vi "sub vi - AI USB4704 (3)  Create Task v2.vi"(0 "Task In 0":dbl, 5 "Task In 1":dbl, 7 "Task In 2":dbl) -> (4 "TASK USB 0":i32, 6 "TASK USB 1":i32, 8 "TASK USB 2":i32, 14 "AI Task Er":bool, 15 "error array":errorcluster[](array[cluster]))   [LabVIEW 2017]
uses:
  <userlib>/DAQNavi Polymorphic VI/create/DAQNavi Create Channel(AI-Voltage).vi
  <userlib>/DAQNavi Polymorphic VI/configure/timing/DAQNavi Timing(Convert Clock).vi
  <userlib>/DAQNavi Polymorphic VI/configure/DAQNavi Get Property/AI/DAQNaviGet_AI_ConvertClock_Rate.vi
panel:
  in  "Tab Control":enum32{"Tasks In", "USB #0", "USB #1", "USB #2"}(tab)
  out "physical channels 0":string="DemoDevice,BID#0/ai0:1" caption="property value"
  out "value range 0":string="+/- 5 V" caption="property value"
  out "convert rate 0":dbl
  out "physical channels 1":string="DemoDevice,BID#0/ai0:1" caption="property value"
  out "value range  1":string="+/- 5 V" caption="property value"
  out "convert rate 1":dbl
  out "physical channels 2":string="DemoDevice,BID#0/ai0:1" caption="property value"
  out "value range  2":string="+/- 5 V" caption="property value"
  out "convert rate 2":dbl
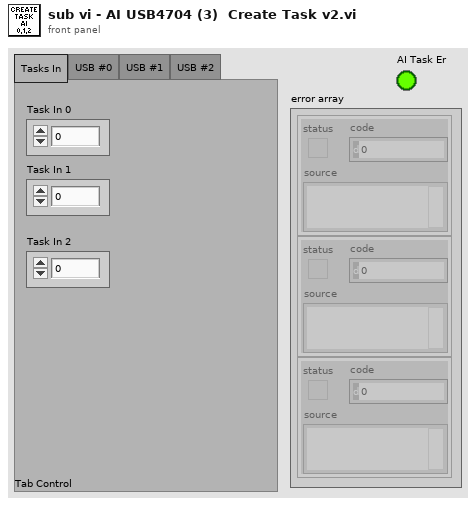
[diagram p1: front panel]
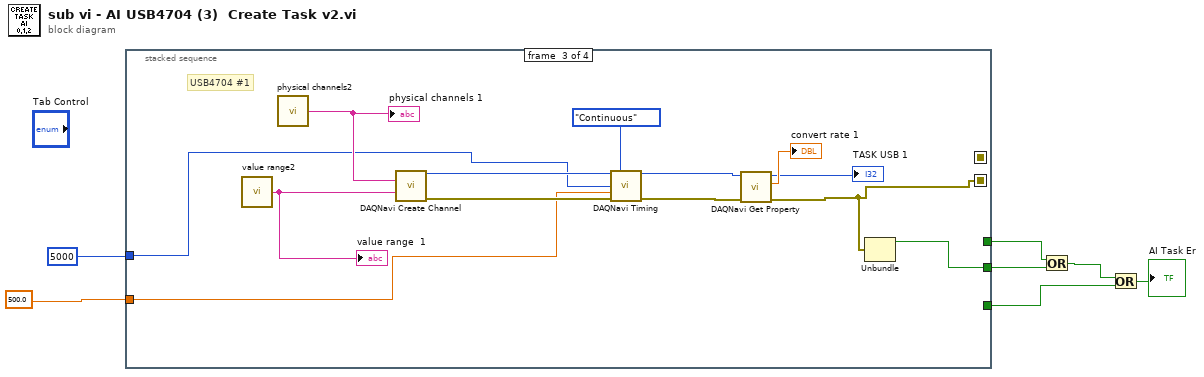
[diagram p0: block diagram]
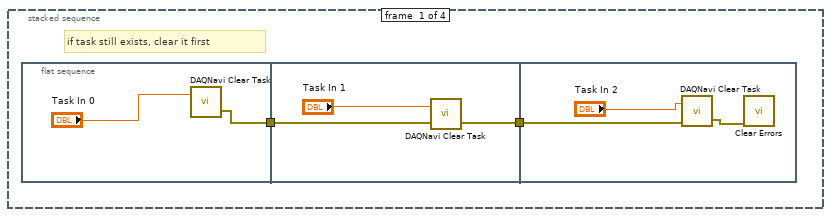
[diagram p2: hidden frame]
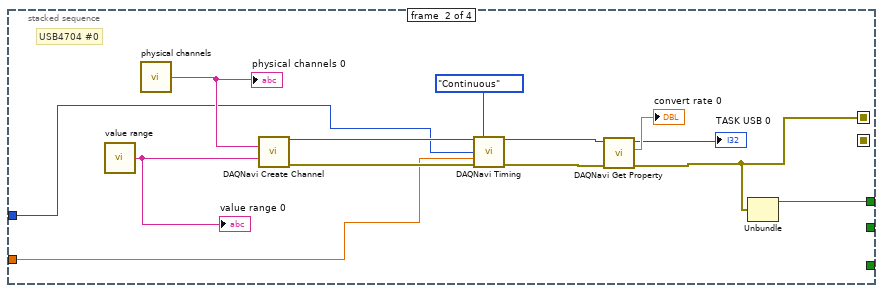
[diagram p3: hidden frame]
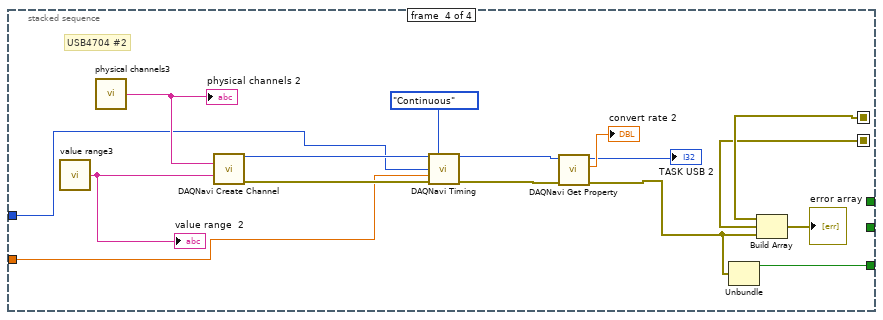
[diagram p4: hidden frame]
diagram:
  n1 = stacked-sequence {
    seq-local: [_ w19 _ _] -> [_ _ _ w50]
    seq-local: [_ _ w32 _] -> [_ _ _ w49]
    tunnel: 5000 -> [_ w21 w34 w47]
    tunnel: 500.0 -> [_ w20 w33 w46]
    tunnel: [_ _ _ w44] -> w4
    tunnel: [_ w18 _ _] -> w3
    tunnel: [_ _ w31 _] -> w2
    frame #0 {
      # "if task still exists, clear it first"
      n2 = flat-sequence {
        tunnel: [w11] -> w9
        tunnel: w9 -> [w14]
        tunnel: [w13] -> w8
        tunnel: w8 -> [w17]
        frame #0 {
          n3 = call <userlib>:"DAQNavi Clear Task.vi"("task in"="Task In 0") -> ("error out"=w11:errorcluster)  [unwired: 2 in]
        }
        frame #1 {
          n4 = call <userlib>:"DAQNavi Clear Task.vi"("error in (no error)"=w14, "task in"="Task In 1") -> ("error out"=w13:errorcluster)  [unwired: 1 in]
        }
        frame #2 {
          n5 = call <userlib>:"DAQNavi Clear Task.vi"("error in (no error)"=w17, "task in"="Task In 2") -> ("error out"=w16:errorcluster)  [unwired: 1 in]
          n6 = call <vilib>:"Clear Errors.vi"("error in (no error)"=w16) -> ()  [unwired: 5 in, 2 out]
        }
      }
    }
    frame #1 {
      # "USB4704 #0"
      n7 = call "value range"() -> ("property value"=w30:string)  [unwired: 1 out]
      "value range 0" <- w30
      n8 = call "physical channels"() -> ("property value"=w29:string)  [unwired: 1 out]
      "physical channels 0" <- w29
      n9 = call-poly <userlib>:"DAQNavi Create Channel.vi"("physical channels"=w29, "value range"=w30) -> ("task out"=w23:i32, "error out"=w24:errorcluster)  [unwired: 3 in, 9 out]
      n10 = call-poly <userlib>:"DAQNavi Timing.vi"("task in"=w23, "sample mode"=enum16{"Finite", "Continuous"}."Continuous", "rate"=w21, "samples per channel"=w20, "error in (no error)"=w24) -> ("task out"=w26:i32, "error out"=w27:errorcluster)  [unwired: 1 in, 8 out]
      n11 = call-poly <userlib>:"DAQNavi Get Property.vi"("error in (no error)"=w27, "task in"=w26) -> ("error out"=w19:errorcluster, "rate"=→"convert rate 0":dbl, "task out"=→"TASK USB 0":i32)  [unwired: 7 out]
      n12 = Unbundle(w19) -> ("status"=w18:bool)  [unwired: 2 out]
    }
    frame #2 {
      # "USB4704 #1"
      n13 = call "value range2"() -> ("property value"=w43:string)  [unwired: 1 out]
      "value range  1" <- w43
      n14 = call "physical channels2"() -> ("property value"=w42:string)  [unwired: 1 out]
      "physical channels 1" <- w42
      n15 = call-poly <userlib>:"DAQNavi Create Channel.vi"("physical channels"=w42, "value range"=w43) -> ("task out"=w36:i32, "error out"=w37:errorcluster)  [unwired: 3 in, 9 out]
      n16 = call-poly <userlib>:"DAQNavi Timing.vi"("task in"=w36, "sample mode"=enum16{"Finite", "Continuous"}."Continuous", "rate"=w34, "samples per channel"=w33, "error in (no error)"=w37) -> ("task out"=w39:i32, "error out"=w40:errorcluster)  [unwired: 1 in, 8 out]
      n17 = call-poly <userlib>:"DAQNavi Get Property.vi"("error in (no error)"=w40, "task in"=w39) -> ("error out"=w32:errorcluster, "rate"=→"convert rate 1":dbl, "task out"=→"TASK USB 1":i32)  [unwired: 7 out]
      n18 = Unbundle(w32) -> ("status"=w31:bool)  [unwired: 2 out]
    }
    frame #3 {
      # "USB4704 #2"
      n19 = call "value range3"() -> ("property value"=w59:string)  [unwired: 1 out]
      "value range  2" <- w59
      n20 = call "physical channels3"() -> ("property value"=w58:string)  [unwired: 1 out]
      "physical channels 2" <- w58
      n21 = call-poly <userlib>:"DAQNavi Create Channel.vi"("physical channels"=w58, "value range"=w59) -> ("task out"=w52:i32, "error out"=w53:errorcluster)  [unwired: 3 in, 9 out]
      n22 = call-poly <userlib>:"DAQNavi Timing.vi"("task in"=w52, "sample mode"=enum16{"Finite", "Continuous"}."Continuous", "rate"=w47, "samples per channel"=w46, "error in (no error)"=w53) -> ("task out"=w55:i32, "error out"=w56:errorcluster)  [unwired: 1 in, 8 out]
      n23 = call-poly <userlib>:"DAQNavi Get Property.vi"("error in (no error)"=w56, "task in"=w55) -> ("error out"=w45:errorcluster, "rate"=→"convert rate 2":dbl, "task out"=→"TASK USB 2":i32)  [unwired: 7 out]
      n24 = Unbundle(w45) -> ("status"=w44:bool)  [unwired: 2 out]
      n25 = Build Array(w50, w49, w45) -> (→"error array":errorcluster[])
    }
  }
  n26 = Or(x=w3, y=w2) -> (x .or. y?=w5:bool)
  n27 = Or(x=w5, y=w4) -> (x .or. y?=→"AI Task Er":bool)
